vi "CheckRange.vi"(10 "Range":T2, 11 "value":dbl) -> (3 "OutOfRange":T1)   [LabVIEW 2019]
uses:
  TypeDef/Range.ctl
  TypeDef/OutOfRange.ctl
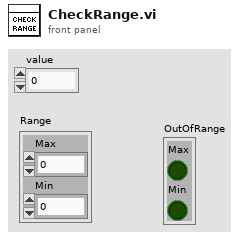
[diagram p1: front panel]
types:
  T1 = typedef "OutOfRange.ctl" = cluster{"Max":bool, "Min":bool}
  T2 = typedef "Range.ctl" = cluster{"Max":dbl, "Min":dbl}
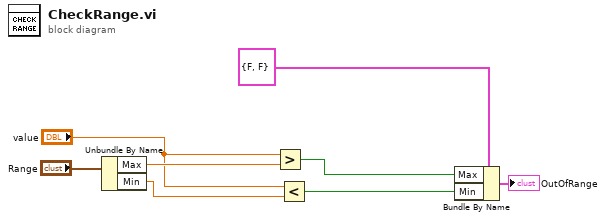
[diagram p0: block diagram]
diagram:
  n1 = Unbundle By Name("Range") -> ("Max"=w7:dbl, "Min"=w4:dbl)
  n2 = Greater?(x="value", y=w7) -> (0:w5:bool)
  n3 = Less?(x="value", y=w4) -> (x < y?=w2:bool)
  n4 = Bundle By Name(cluster=T1 {"Max"=FALSE, "Min"=FALSE} ("OutOfRange"), "Max"=w5, "Min"=w2) -> (→"OutOfRange":T1)
